vi "断电保存全局.vi"() -> ()   [LabVIEW 2016, in "中水三立SQL数据传输.lvlib"]
panel:
  in  "数据查表起始时间":cluster{"dbo.LS_Data":string}
  in  "配置信息":T1
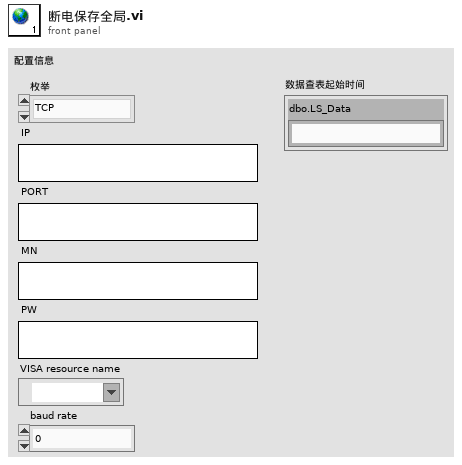
[diagram p1: front panel]
types:
  T1 = cluster{"枚举":enum16{"TCP", "serial"}, "IP":string, "PORT":string, "MN":string, "PW":string, "VISA resource name":refnum<visa-resource-name>, "baud rate":u32}
diagram:
